vi "nominal run start.vi"(8 "error in (no error)":errorcluster, 10 "out_millis":dbl, 11 "run":i32) -> (0 "error out":errorcluster, 2 "out_millis out":dbl, 3 "function return":i32)   [LabVIEW 2020, in "client.lvlib"]
doc: "int32_t nominal_run_start(int32_t run, double *out_millis);"
uses:
  client.lvlib
  bin/nominalClient_64.dll
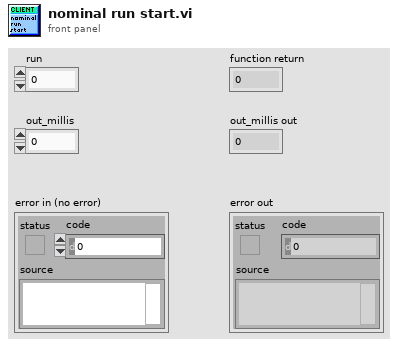
[diagram p1: front panel]
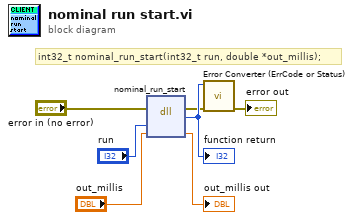
[diagram p0: block diagram]
diagram:
  # "int32_t nominal_run_start(int32_t run, double *out_millis);"
  n1 = dll-call lib="C:/code/labview-client-rs/lv_src/bin/nominalClient_*.*" fn="nominal_run_start"(error in="error in (no error)", "run"="run", "out_millis"="out_millis") -> (error out=w2:errorcluster, w7:i32, "out_millis"=→"out_millis out":dbl)  [unwired: 3 in, 1 out]
  "function return" <- w7
  n2 = call "Error Converter (ErrCode or Status).vi"("error in (no error)"=w2, "error code"=w7) -> ("error out"=→"error out":errorcluster)  [unwired: 9 in]
